vi "ModbusTxFIFOUpdateLoop.vi"(11 "Modbus Port Settings":T1={"TxPort"="ModbusPort1Tx", "TxDataFIFO"="ModbusPort1TxFIFO", "TxInternalDataFIFO"="ModbusPort1TxInternalFIFO", "TxHealthAndStatusFIFO"="ModbusPort1TxHealthAndStatusFIFO", "RxPort"="ModbusPort1Rx", "RxDataFIFO"="ModbusPort1RxFIFO", "RxHealthAndStatusFIFO"="ModbusPort1RxHealthAndStatusFIFO", "WaitForRxFrameRegister"="ModbusPort1WaitForRxControl", "BaseHealthAndStatusAddress"=0, "IRQAddress"=0, "TriggerIRQRegister"="ModbusPort1IRQControl", "SoftwareControlledTrigger"="ModbusSoftwareControlledTrigger", "TimestampRegister"="TimestampRegister", "TxTimestampFIFO"="ModbusPort1TimestampFIFO"}) -> ()   [LabVIEW 2016, in "FPGAModbus.lvlib"]
uses:
  FPGAModbus.lvlib
  DataTypes/ModbusPortSettings.ctl
  <vilib>/Platform/TimedLoop/XDataNode/timing_clust.ctl
  <vilib>/Platform/TimedLoop/XDataNode/nitl_modes.ctl
  <vilib>/Platform/TimedLoop/XDataNode/wakeup.ctl
  DataTypes/ModbusTxInstruction.ctl
  DataTypes/ModbusTxInstructionTypes.ctl
  Common_FPGA_HealthAndStatus/DataTypes/HealthAndStatusUpdateMode.ctl
  <vilib>/rvi/Emulation/niFpgaSctlEmulationGetInTimedLoop.vi
  <vilib>/rvi/Emulation/niFpgaEmulationReportErrorSimple.vi
  <vilib>/rvi/Emulation/niFpgaGetClockAttributes.vi
  <vilib>/rvi/Emulation/niFpgaCriticalErrorInLSC.vi
  <vilib>/rvi/DataTransferAndStorage/Container/Common/niFpgaContainerExecOnDevCompGetState.vi
  <vilib>/rvi/Emulation/niFpgaEmulationIsFPGAContextNoSignature.vi
  <vilib>/rvi/errors/niFpgaSetErrorForExecOnDevCompSimple.vi
  <vilib>/rvi/eio/common/nirviEmuReportErrorAndStop.vi
  <vilib>/rvi/DataTransferAndStorage/Container/Common/niFpgaContainerGetUniqueNameForEmu.vi
  <vilib>/rvi/FIFO/Fifo_Resource/nirvififoEmulationSetSize.vi
  <vilib>/rvi/FIFO/Fifo_Resource/nirviFifoEmulationQueueMgr.vi
  <instcachedir>/0/nirviFifoEmulationQueueMgr_E5CAEC123FF24DC58D834DCA3CDAA9B5.lvgen/nirviFifoEmulationQueueMgr_E5CAEC123FF24DC58D834DCA3CDAA9B5_002.vi
  <vilib>/rvi/FIFO/Fifo_Resource/nirvififoEmulationDetermineInputValidOut.vi
  <vilib>/rvi/FIFO/Fifo_Resource/nirvififoEmulationCreateLock.vi
  <vilib>/rvi/Emulation/niFpgaProcessEmulError.vi
  <vilib>/rvi/FIFO/Fifo_Resource/nirvififoEmulationObtainLock.vi
  <vilib>/rvi/FIFO/Fifo_Resource/nirvififoEmulationReleaseLock.vi
  <vilib>/rvi/occurrence/nirviWaitOnOccurrenceBase.vi
  <vilib>/rvi/errors/nirviReportUnexpectedCaseInternalError.vi
  <vilib>/rvi/errors/nirviReportUnexpectedCaseInternalError (U32).vi
  <vilib>/Utility/error.llb/Clear Errors.vi
  <vilib>/rvi/interface/RandomDataEmulation/niFpgaRandomDataHandleErrors.vi
  <instcachedir>/0/nirviFifoEmulationQueueMgr_E5CAEC123FF24DC58D834DCA3CDAA9B5.lvgen/nirviFifoEmulationQueueMgr_E5CAEC123FF24DC58D834DCA3CDAA9B5_010.vi
  <vilib>/Platform/TimedLoop/XDataNode/XDataNode.xnode
  <vilib>/rvi/DataTransferAndStorage/Container/XNode/niFpgaContainer.xnode
  <vilib>/rvi/FIFO/Fifo_Resource/niFpgaFifoEmulationRefIn.vi
  <vilib>/Platform/TimedLoop/XDataNode/XDNodeRunTimeDep.lvlib
  Common_FPGA_HealthAndStatus/FPGAHealthAndStatus.lvlib
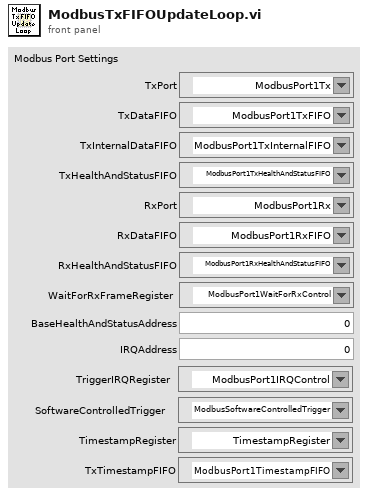
[diagram p1: front panel]
types:
  T1 = typedef "FPGAModbus.lvlib/ModbusPortSettings.ctl" = cluster{"TxPort":refnum<k21>, "TxDataFIFO":refnum<k21>, "TxInternalDataFIFO":refnum<k21>, "TxHealthAndStatusFIFO":refnum<k21>, "RxPort":refnum<k21>, "RxDataFIFO":refnum<k21>, "RxHealthAndStatusFIFO":refnum<k21>, "WaitForRxFrameRegister":refnum<k21>, "BaseHealthAndStatusAddress":u32, "IRQAddress":u8, "TriggerIRQRegister":refnum<k21>, "SoftwareControlledTrigger":refnum<k21>, "TimestampRegister":refnum<k21>, "TxTimestampFIFO":refnum<k21>}
  T2 = typedef "XDNodeRunTimeDep.lvlib/timing_clust.ctl" = cluster{"Expected End [f-1]":u64, "Actual End [f-1]":u64, "Finished Late? [f-1]":bool, "Expected End [i-1]":u64, "Actual End [i-1]":u64, "Finished Late? [i-1]":bool, "Expected Start [i]":u64, "Actual Start [i]":u64, "Expected Start [f]":u64, "Actual Start [f]":u64, "Source Name":string, "Structure Name":string, "Period":i64, "Deadline":i64, "Offset":i64, "Start":i64, "Priority":i32, "Timeout":i32, "Mode":T3, "Wakeup Reason":T4, "Error":errorcluster, "Source Type":string, "Secondary Source Type":string, "Global End Time":u64, "Global Start Time":u64, "Frame Duration":u64, "Iteration Duration":u64, "Assigned CPU":i32, "I/O Scan Engine Mode":u32}
  T3 = typedef "XDNodeRunTimeDep.lvlib/nitl_modes.ctl" = enum32{"No Change", "Process missed periods, maintain original phase", "Discard missed periods, maintain original phase", "Process missed periods, ignore original phase", "Discard missed periods, ignore original phase"}
  T4 = typedef "XDNodeRunTimeDep.lvlib/wakeup.ctl" = enum32{"Normal", "Aborted", "Asynchronous wakeup", "Timing source error", "Timed loop error", "Timeout"}
  T5 = typedef "FPGAModbus.lvlib/ModbusTxInstruction.ctl" = cluster{"InstructionType":T6, "Data":u16}
  T6 = typedef "FPGAModbus.lvlib/ModbusTxInstructionTypes.ctl" = enum8{"NOP", "WriteByte", "EndOfFrame", "PushTimestamp", "DelayMicroseconds", "DelayMilliseconds", "WaitForRxFrame", "TriggerIRQ", "WaitForTrigger", "WaitForLongRxFrame"}
  T7 = typedef "FPGAHealthAndStatus.lvlib/HealthAndStatusUpdateMode.ctl" = enum8{"NOP", "Set", "Add", "Subtract", "Or"}
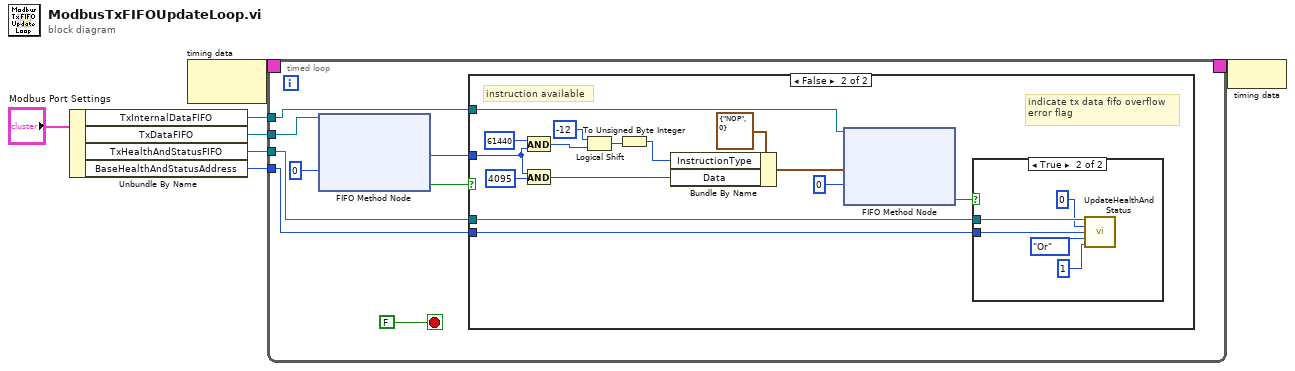
[diagram p0: block diagram]
diagram:
  n1 = Unbundle By Name("Modbus Port Settings") -> ("TxInternalDataFIFO"=w4:refnum<k21>, "TxDataFIFO"=w5:refnum<k21>, "TxHealthAndStatusFIFO"=w2:refnum<k21>, "BaseHealthAndStatusAddress"=w1:u32)
  n2 = node-c288() -> (w7:T2)  [unwired: 1 in]
  n3 = timed-loop {
    timing: w7 -> [_]
    timing-out: [_] -> w6
    tunnel: w4 -> [w9]
    tunnel: w5 -> [w8]
    tunnel: w2 -> [w12]
    tunnel: w1 -> [w11]
    stop <- FALSE stop-if-true
    n4 = xnode ("FIFO Method Node")("Timeout"=0, "FIFO In"=w8) -> ("Element"=w13:u16, "Timed Out?"=w14:bool)  [unwired: 1 out]
    n5 = case shown="False" w14 {
      tunnel: w13 -> [_ w24]
      tunnel: w9 -> [_ w19]
      tunnel: w12 -> [_ w22]
      tunnel: w11 -> [_ w21]
      frame True {
        # "no instruction available"
      }
      frame False {
        # "indicate tx data fifo overflow\nerror flag"
        # "instruction available"
        n6 = And(x=u16 61440 ("y"), y=w24) -> (x .and. y?=w29:u16)
        n7 = And(x=w24, y=u16 4095) -> (x .and. y?=w26:u16)
        n8 = Logical Shift(y=i16 -12, x=w29) -> (x << y=w27:u16)
        n9 = To Unsigned Byte Integer(number=w27) -> (unsigned 8bit integer=w25:u8)
        n10 = Bundle By Name(cluster=T5 {"InstructionType"=enum."NOP", "Data"=0} ("Tx Instruction"), "InstructionType"=w25, "Data"=w26) -> (w16:T5)
        n11 = xnode ("FIFO Method Node")("Element"=w16, "Timeout"=0, "FIFO In"=w19) -> ("Timed Out?"=w17:bool)  [unwired: 1 out]
        n12 = case shown="True" w17 {
          tunnel: w22 -> [_ w35]
          tunnel: w21 -> [_ w34]
          frame False {
          }
          frame True {
            n13 = call "UpdateHealthAndStatus.vi"("InternalHealthAndStatusFIFO"=w35, "AddressOffset"=u32 0 ("Address Offset"), "BaseAddress"=w34, "HealthAndStatusUpdateMode"=HealthAndStatusUpdateMode."Or" ("Telemetry Update Mode"), "Data"=u64 1) -> ()  [unwired: 11 in]
          }
        }
      }
    }
  }
  n14 = node-c288(w6) -> ()
